vi "Motor_Stop.vi"(8 "error in (no error)":errorcluster, 11 "Lifter_motor in":refnum<class "Lifter_motor.lvclass">) -> (0 "error out":errorcluster, 2 "Driver ACK?":bool, 3 "Lifter_motor out":refnum<class "Lifter_motor.lvclass">)   [LabVIEW 2019, in "Lifter_motor.lvclass"]
uses:
  Lifter_motor.lvclass
  Lifter_motor.lvclass/Lifter_motor.ctl
  TCP Class/LifterTCP.lvclass
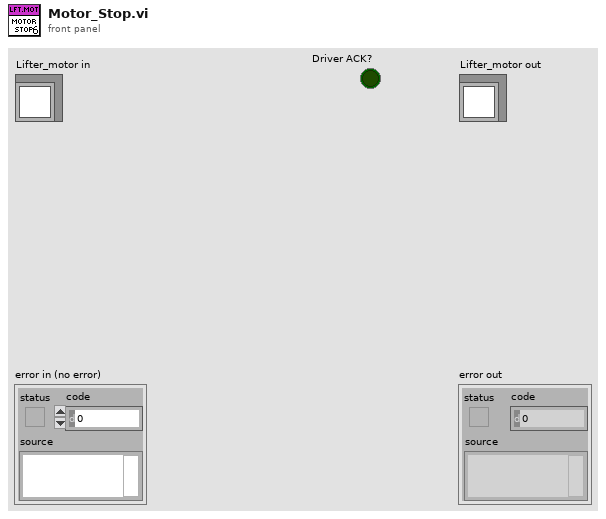
[diagram p1: front panel]
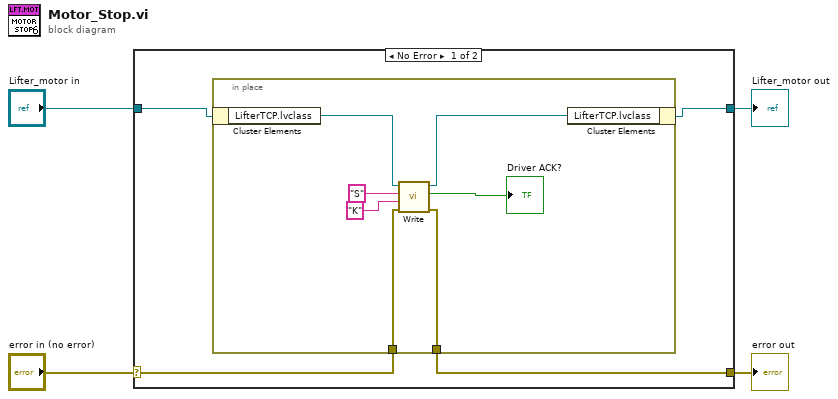
[diagram p0: block diagram]
diagram:
  n1 = case shown="No Error" "error in (no error)" {
    selector: "error in (no error)" -> [w6 w17]
    tunnel: [w5 w17] -> w3
    tunnel: [w7 w16] -> w1
    tunnel: "Lifter_motor in" -> [w8 w16]
    frame No Error {
      n2 = in-place {
        in-place-border: w6 -> [w11]
        in-place-border: [w10] -> w5
        n3 = in-place-cluster #1(w8) -> ("LifterTCP.lvclass"=w15:refnum<class "LifterTCP.lvclass">)
        n4 = call "Write.vi"("error in (no error)"=w11, "Parameter 2"="K", "Parameter 1"="S", "LifterTCP in"=w15) -> ("error out"=w10:errorcluster, "Driver ACK?"=→"Driver ACK?":bool, "LifterTCP out"=w14:refnum<class "LifterTCP.lvclass">)  [unwired: 5 in]
        n5 = in-place-cluster #1("LifterTCP.lvclass"=w14) -> (w7:refnum<class "Lifter_motor.lvclass">)
      }
    }
    frame Error {
    }
  }
  "error out" <- w3
  "Lifter_motor out" <- w1
